vi "OAT Demodulation with Decimation (N Freq, N Ch).vi"(0 "x[n]":dbl[][](array[numeric]) format="%.2f", 1 "reset? (True)":bool=TRUE, 2 "zero delay? (F)":bool, 5 "fs":dbl=1.0 format="%.2f", 9 "fc [Hz]":dbl[](array[numeric])=[0.0] format="%.2f", 11 "decimation factor":i32=16, 12 "stop band attenuation":u16(ring) items=["72 dB", "96 dB", "120 dB"], 14 "phase setting":T1) -> (3 "lags":i32, 4 "magnitudes (RMS)":dbl[][][](array[numeric]) format="%.2f", 6 "phase lag":dbl[][][](array[numeric]) format="%.2f", 10 "new fs [Hz]":dbl format="%.2f", 15 "error out":errorcluster)   [LabVIEW 2017, in "SoundVib_Resampling.lvlib"]
uses:
  <vilib>/addons/Sound and Vibration/Order Analysis/Resample Order Tracking/SoundVib_Resampling.lvlib
  <vilib>/addons/Sound and Vibration/Order Analysis/Misc/OAT Convert Phase (N Channels).vi
  <vilib>/Analysis/NI_AALPro.lvlib
panel:
  # "Demodulation"
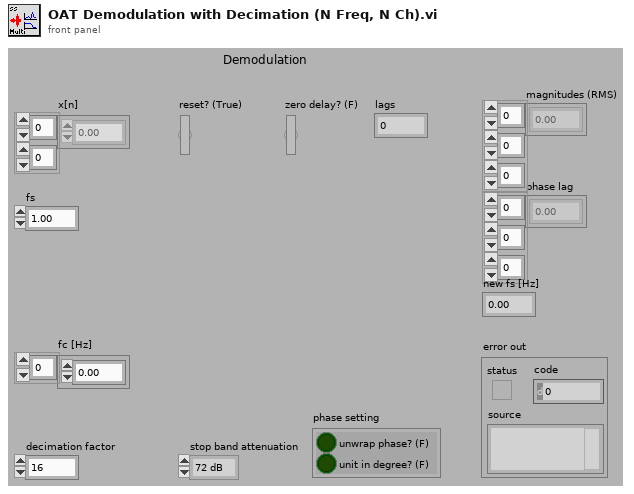
[diagram p1: front panel]
types:
  T1 = cluster{"unwrap phase? (F)":bool, "unit in degree? (F)":bool}
  T2 = typedef "OAT Decimation Filter.ctl" = cluster{"coefficients":dbl[], "factor":i32}
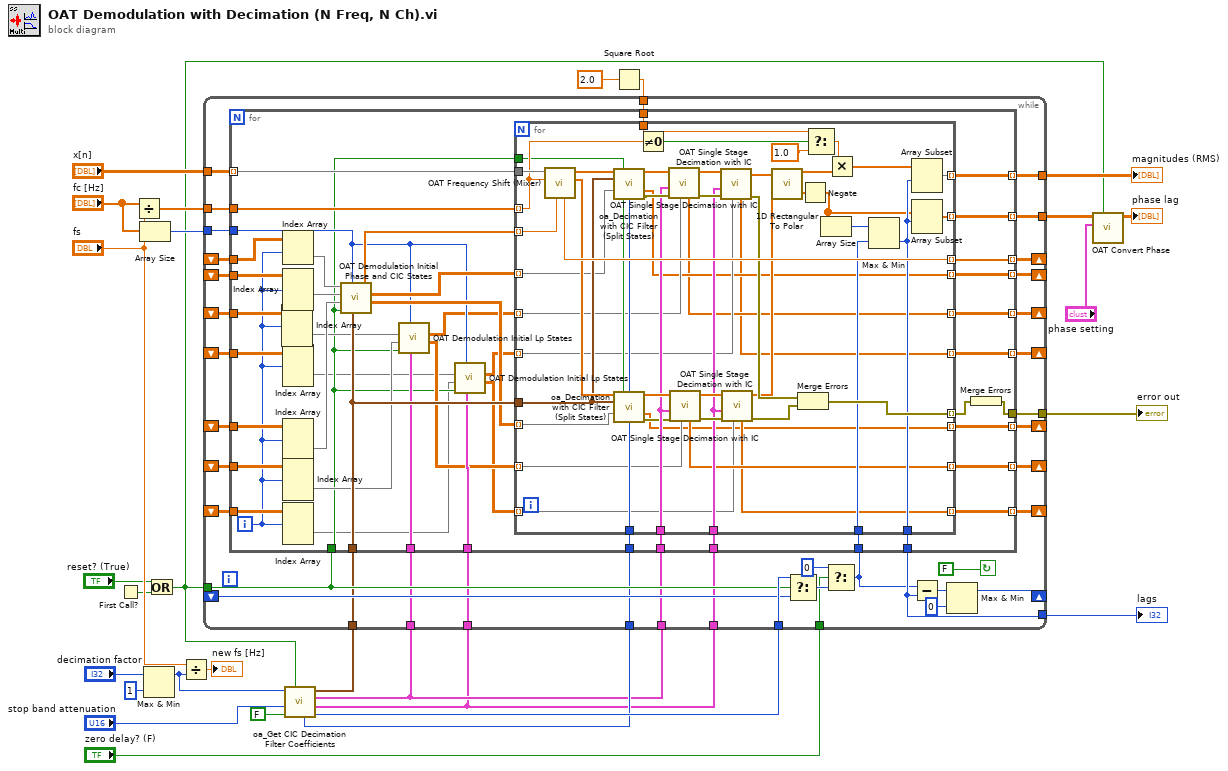
[diagram p0: block diagram]
diagram:
  n1 = First Call?() -> (First Call?: T/F=w17:bool)
  n2 = Divide(x="fc [Hz]", y="fs") -> (x/y=w28:dbl[])
  n3 = Array Size(array="fc [Hz]") -> (size(s)=w27:i32)
  n4 = Max & Min(x="decimation factor", y=1) -> (max(x,y)=w4:i32)  [unwired: 1 out]
  n5 = Or(x="reset? (True)", y=w17) -> (x .or. y?=w9:bool)
  n6 = Divide(x="fs", y=w4) -> (x/y=→"new fs [Hz]":dbl)
  n7 = call <vilib>:"oa_Get CIC Decimation Filter Coefficients.vi"("reset? (True)"=w9, "alias protect in final transition"=FALSE, "stop band attenuation"="stop band attenuation", "decimation/interpolation factor"=w4) -> ("delay"=w10:i32, "lp filter settings"=w1:T2, "compensation filter settings"=w2:T2, "CIC Settings"=w8:cluster{"Numeric":i32, i32, i32}, "interpolation factor"=w7:i32)  [unwired: 3 in]
  n8 = Square Root(x=2.0) -> (sqrt(x)=w25:dbl)
  n9 = while {
    tunnel: w25 -> [w57]
    tunnel: w27 -> [w58]
    shift-left: _ -> [w60]
    shift-right: [w61] -> _
    tunnel: w9 -> [w52]
    shift-left: _ -> [w59]
    shift-right: [w62] -> _
    shift-left: _ -> [w63]
    shift-right: [w64] -> _
    tunnel: w28 -> [w66]
    tunnel: "x[n]" -> [w67]
    tunnel: [w56] -> w12
    tunnel: [w55] -> w24
    tunnel: [w54] -> w15
    tunnel: [w50] -> w14
    shift-right: [w47] -> _
    shift-left: _ -> [w51]
    tunnel: w10 -> [w53]
    tunnel: w8 -> [w46]
    tunnel: w7 -> [w45]
    tunnel: "zero delay? (F)" -> [w41]
    shift-right: [w40] -> _
    shift-left: _ -> [w39]
    shift-right: [w38] -> _
    shift-left: _ -> [w37]
    tunnel: w2 -> [w36]
    tunnel: w1 -> [w35]
    tunnel: w2 -> [w34]
    tunnel: w1 -> [w33]
    shift-right: [w32] -> _
    shift-left: _ -> [w29]
    shift-right: [w31] -> _
    shift-left: _ -> [w30]
    stop <- FALSE continue-if-true
    n10 = Select(t=w53, s=w52, f=w51) -> (s? t:f=w43:i32)
    n11 = Select(t=0 ("x"), s=w41, f=w43) -> (s? t:f=w42:i32)
    n12 = for {
      tunnel: w67 -> [w113] mode=indexing
      tunnel: w66 -> [w112]
      tunnel: [w111] -> w64 mode=indexing
      tunnel: w63 -> [w99]
      tunnel: [w110] -> w62 mode=indexing
      tunnel: [w109] -> w61 mode=indexing
      tunnel: w60 -> [w100]
      tunnel: w59 -> [w83]
      tunnel: w58 -> [w86]
      tunnel: w57 -> [w107]
      tunnel: [w106] -> w56 mode=indexing
      tunnel: [w105] -> w55 mode=indexing
      tunnel: [w103] -> w54
      tunnel: w52 -> [w74]
      tunnel: w42 -> [w102]
      tunnel: [w101] -> w50
      tunnel: w46 -> [w98]
      tunnel: w45 -> [w97]
      tunnel: [w94] -> w40 mode=indexing
      tunnel: w39 -> [w93]
      tunnel: [w91] -> w38 mode=indexing
      tunnel: w37 -> [w90]
      tunnel: w36 -> [w87]
      tunnel: w35 -> [w85]
      tunnel: w34 -> [w80]
      tunnel: w33 -> [w79]
      tunnel: [w76] -> w32 mode=indexing
      tunnel: [w73] -> w31 mode=indexing
      tunnel: w30 -> [w72]
      tunnel: w29 -> [w70]
      i -> [w69]
      n13 = Index Array(array=w83, index (dim 0)=w69) -> (element=w82:dbl[][])  [unwired: 2 in]
      n14 = Index Array(array=w100, index (row)=w69) -> (element=w96:dbl[])  [unwired: 1 in]
      n15 = Index Array(array=w93, index (dim 0)=w69) -> (element=w92:dbl[][])  [unwired: 2 in]
      n16 = Index Array(array=w72, index (dim 0)=w69) -> (element=w71:dbl[][])  [unwired: 2 in]
      n17 = Index Array(array=w90, index (dim 0)=w69) -> (element=w89:dbl[][])  [unwired: 2 in]
      n18 = Index Array(array=w99, index (dim 0)=w69) -> (element=w75:dbl[][])  [unwired: 2 in]
      n19 = Index Array(array=w70, index (dim 0)=w69) -> (element=w68:dbl[][])  [unwired: 2 in]
      n20 = call <vilib>:"OAT Demodulation Initial Phase and CIC States.vi"("CIC filter settings"=w98, "num of orders"=w86, "reset? (True)"=w74, "CIC Image in"=w89, "CIC Real in"=w92, "start phase in"=w96) -> ("CIC Image"=w88:dbl[][], "CIC Real"=w95:dbl[][], "start phase out"=w108:dbl[])  [unwired: 3 in]
      n21 = call <vilib>:"OAT Demodulation Initial Lp States.vi"("filter"=w87, "num of orders"=w86, "reset? (True)"=w74, "Lp Image in"=w75, "Lp Real in"=w82) -> ("Lp Image"=w78:dbl[][], "Lp Real"=w84:dbl[][])  [unwired: 5 in]
      n22 = call <vilib>:"OAT Demodulation Initial Lp States.vi"("filter"=w85, "num of orders"=w86, "reset? (True)"=w74, "Lp Image in"=w68, "Lp Real in"=w71) -> ("Lp Image"=w77:dbl[][], "Lp Real"=w81:dbl[][])  [unwired: 5 in]
      n23 = for {
        tunnel: w113 -> [w160]
        tunnel: w112 -> [w149] mode=indexing
        tunnel: [w162] -> w109 mode=indexing
        tunnel: w108 -> [w126] mode=indexing
        tunnel: w107 -> [w147]
        tunnel: [w153] -> w106 mode=indexing
        tunnel: [w154] -> w105 mode=indexing
        tunnel: [w156] -> w104 mode=indexing
        tunnel: w102 -> [w151]
        tunnel: [w150] -> w101
        tunnel: w74 -> [w144]
        tunnel: w98 -> [w142]
        tunnel: w97 -> [w141]
        tunnel: w80 -> [w133]
        tunnel: w79 -> [w127]
        tunnel: w95 -> [w125] mode=indexing
        tunnel: [w122] -> w94 mode=indexing
        tunnel: w84 -> [w124] mode=indexing
        tunnel: [w121] -> w110 mode=indexing
        tunnel: w81 -> [w123] mode=indexing
        tunnel: [w120] -> w73 mode=indexing
        tunnel: w88 -> [w119] mode=indexing
        tunnel: [w114] -> w91 mode=indexing
        tunnel: w78 -> [w118] mode=indexing
        tunnel: [w117] -> w111 mode=indexing
        tunnel: w77 -> [w116] mode=indexing
        tunnel: [w115] -> w76 mode=indexing
        n24 = call <vilib>:"OAT Frequency Shift (Mixer).vi"("initial phase"=w126, "fc"=w149, "X"=w160) -> ("imaginary"=w159:dbl[], "real"=w158:dbl[], "final phase"=w162:dbl)  [unwired: 6 in]
        n25 = call <vilib>:"oa_Decimation with CIC Filter (Split States).vi"("x[n]"=w158, "reset? (True)"=w144, "CIC decimation setting"=w142, "CIC state"=w125, "interpolation factor"=w141) -> ("x[n] out"=w140:dbl[], "final CIC state"=w122:dbl[], "error out"=w137:errorcluster)  [unwired: 8 in]
        n26 = call <vilib>:"oa_Decimation with CIC Filter (Split States).vi"("x[n]"=w159, "reset? (True)"=w144, "CIC decimation setting"=w142, "CIC state"=w119, "interpolation factor"=w141) -> ("x[n] out"=w134:dbl[], "final CIC state"=w114:dbl[], "error out"=w130:errorcluster)  [unwired: 8 in]
        n27 = Not Equal To 0?(x=w149) -> (x != 0?=w148:bool)
        n28 = call <vilib>:"OAT Single Stage Decimation with IC.vi"("initial state"=w124, "error in (no error)"=w137, "filter"=w133, "X"=w140) -> ("error out"=w136:errorcluster, "Y"=w138:dbl[], "final state"=w121:dbl[])  [unwired: 5 in]
        n29 = call <vilib>:"OAT Single Stage Decimation with IC.vi"("initial state"=w118, "error in (no error)"=w130, "filter"=w133, "X"=w134) -> ("error out"=w132:errorcluster, "Y"=w131:dbl[], "final state"=w117:dbl[])  [unwired: 5 in]
        n30 = call <vilib>:"OAT Single Stage Decimation with IC.vi"("initial state"=w123, "error in (no error)"=w136, "filter"=w127, "X"=w138) -> ("error out"=w135:errorcluster, "Y"=w139:dbl[], "final state"=w120:dbl[])  [unwired: 5 in]
        n31 = call <vilib>:"OAT Single Stage Decimation with IC.vi"("initial state"=w116, "error in (no error)"=w132, "filter"=w127, "X"=w131) -> ("error out"=w129:errorcluster, "Y"=w128:dbl[], "final state"=w115:dbl[])  [unwired: 5 in]
        n32 = call <vilib>:"1D Rectangular To Polar.vi"("X"=w139, "Y"=w128) -> ("Magnitude"=w161:dbl[], "Phase"=w157:dbl[])  [unwired: 1 out]
        n33 = Merge Errors(w135, w129) -> (w156:errorcluster)
        n34 = Negate(x=w157) -> (-x=w143:dbl[])
        n35 = Select(t=w147, s=w148, f=1.0) -> (s? t:f=w146:dbl)
        n36 = Array Size(array=w143) -> (size(s)=w152:i32)
        n37 = Multiply(x=w146, y=w161) -> (x*y=w155:dbl[])
        n38 = Max & Min(x=w152, y=w151) -> (min(x,y)=w150:i32)  [unwired: 1 out]
        n39 = Array Subset(array=w155, index=w150) -> (w154:dbl[])  [unwired: 1 in]
        n40 = Array Subset(array=w143, index=w150) -> (w153:dbl[])  [unwired: 1 in]
      }
      n41 = Merge Errors(w104) -> (w103:errorcluster)
    }
    n42 = Subtract(x=w42, y=w50) -> (x-y=w49:i32)
    n43 = Max & Min(x=w49, y=0) -> (max(x,y)=w47:i32)  [unwired: 1 out]
  }
  "error out" <- w15
  "magnitudes (RMS)" <- w24
  "lags" <- w14
  n44 = call-poly <vilib>:"OAT Convert Phase.vi"("reset (TRUE)"=w9, "desired phase setting"="phase setting", "phase in"=w12) -> ("phase out"=→"phase lag":dbl[][][])  [unwired: 8 in]
